vi "DataStream_PC_Create.vi"(11 "Target IP Address (10.58.47.2)":string="10.58.47.2") -> (0 "Error Out":errorcluster, 3 "Stream Ref Out":T1)   [LabVIEW 2023]
uses:
  TypeDefs/Cluster_DataStream_PC Reader Refs.ctl
  <vilib>/dex/Stream Element Allocation Mode.ctl
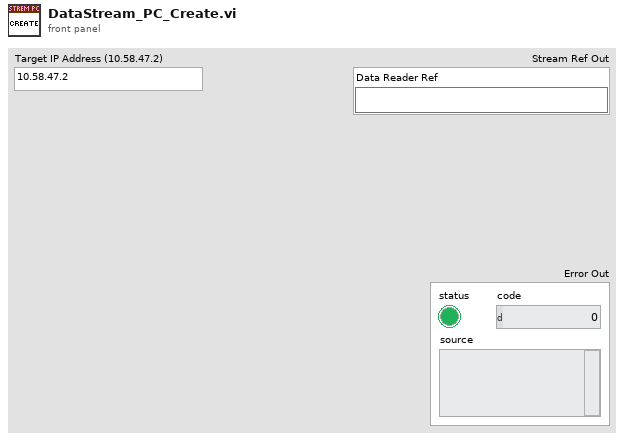
[diagram p1: front panel]
types:
  T1 = typedef "Cluster_DataStream_PC Reader Refs.ctl" = cluster{"Data Reader Ref":refnum<k21>}
  T2 = typedef "Stream Element Allocation Mode.ctl" = u32
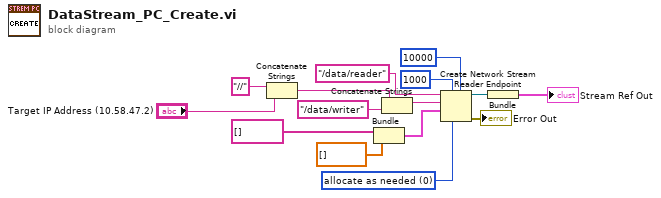
[diagram p0: block diagram]
diagram:
  w15 = T2 0 items=["allocate as needed", "pre-allocate"] ("element allocation mode")
  n1 = Concatenate Strings("//" ("reader url"), "Target IP Address (10.58.47.2)") -> (w8:string)
  n2 = Bundle(string[] [], dbl[] []) -> (w3:cluster{string[], dbl[]})  [unwired: 1 in]
  n3 = Concatenate Strings(w8, "/data/writer" ("reader url")) -> (w13:string)
  n4 = Create Network Stream Reader Endpoint(5:10000 ("timeout in ms (-1)"), 6:w15, 7:1000 ("reader buffer size"), 9:w3, 10:w13, 11:"/data/reader" ("writer name")) -> (0:→"Error Out":errorcluster, 3:w6:refnum<k21>)  [unwired: 1 in]
  n5 = Bundle("writer name"=w6) -> (→"Stream Ref Out":cluster{"writer name":refnum<k21>})  [unwired: 1 in]
